vi "Setup_Environment.vi"() -> (0 "First Time":bool)   [LabVIEW 2022 SP3]
uses:
  File/Setup_Filetype.ctl
  Globals/Meas_global.vi
panel:
  out "error string":string
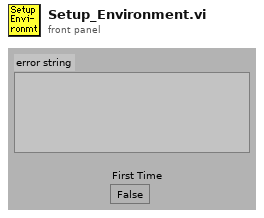
[diagram p1: front panel]
types:
  T1 = typedef "Setup_Filetype.ctl" = enum16{"Measurement Setups", "Calibration Setups", "General", "Results File Plotter Setups", "Speed Calib Tweaks"}
  T2 = cluster{"Start Index":i32, "End Index":i32, "Smoothing":enum16{"Linear", "Logarithmic"}, "Number of smoothed estimates":i32, "X axis":cluster{"Mapping":u16, "Format":u16}, "Y axis":cluster{"Mapping":u16, "Format":u16}, "Use Whole Input Array?":bool}[]
  T3 = cluster{"Start Index":i32, "End Index":i32, "Smoothing":enum16{"Linear", "Logarithmic"}, "Number of smoothed estimates":i32, "X axis":cluster{"Mapping":u16, "Format":u16}, "Y axis":cluster{"Mapping":u16, "Format":u16}, "Use Whole Input Array?":bool}
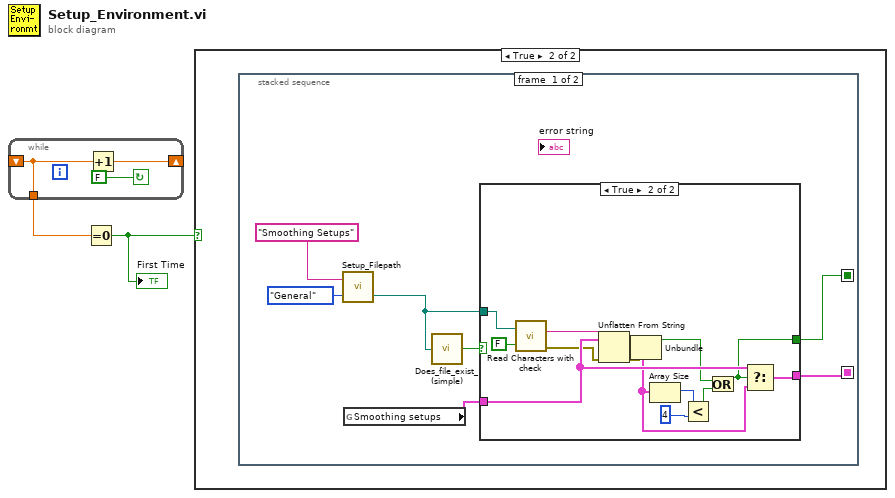
[diagram p0: block diagram]
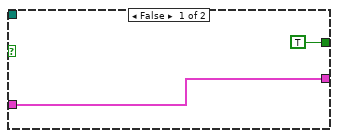
[diagram p3: hidden frame]
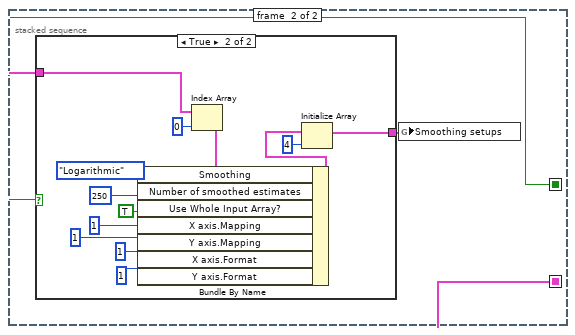
[diagram p4: hidden frame]
diagram:
  n1 = while {
    tunnel: [w5] -> w2
    shift-left: _ -> [w5]
    shift-right: [w4] -> _
    stop <- FALSE continue-if-true
    n2 = Increment(x=w5) -> (x+1=w4:dbl)
  }
  n3 = Equal To 0?(x=w2) -> (x = 0?=w1:bool)
  "First Time" <- w1
  n4 = case shown="True" w1 {
    frame False {
    }
    frame True {
      n5 = stacked-sequence {
        seq-local: [w10 _] -> [_ w30]
        seq-local: [w9 _] -> [_ w29]
        frame #0 {
          n6 = call "Setup_Filepath.vi"("Setup File Type"=Setup_Filetype."General", "Filename in"="Smoothing Setups" ("Substring")) -> ("Filename Out"=w6:path)  [unwired: 1 out]
          n7 = global read "Meas_global.vi" "Smoothing setups"() -> (w11:T2)
          n8 = call "Does_file_exist_(simple).vi"("Pathname"=w6) -> ("exists?"=w12:bool)
          n9 = case shown="True" w12 {
            tunnel: w6 -> [_ w18]
            tunnel: w11 -> [w14 w27]
            tunnel: [TRUE ("err") w20] -> w10
            tunnel: [w14 w26] -> w9
            frame False {
            }
            frame True {
              n10 = call "Read Characters with check.vi"("Call EnFlo Error Handler?"=FALSE, "file (use dialog)"=w18) -> ("error out"=w16:errorcluster, "Read String"=w17:string)
              n11 = Unflatten From String(type=w27, binary string=w17, error in (no error)=w16) -> (value=w21:T2, error out=w19:errorcluster)  [unwired: 3 out]
              n12 = Unbundle(w19) -> ("status"=w22:bool)  [unwired: 2 out]
              n13 = Array Size(array=w21) -> (size(s)=w25:i32)
              n14 = Less?(x=w25, y=4) -> (x < y?=w23:bool)
              n15 = Or(x=w22, y=w23) -> (x .or. y?=w20:bool)
              n16 = Select(t=w27, s=w20, f=w21) -> (s? t:f=w26:T2)
            }
          }
        }
        frame #1 {
          n17 = case shown="True" w30 {
            tunnel: [w31 w41] -> w28
            tunnel: w29 -> [w31 w34]
            frame False {
            }
            frame True {
              n18 = Index Array(array=w34, index=0 ("Index")) -> (element=w42:T3)
              n19 = Bundle By Name(cluster=w42, "Smoothing"=enum16{"Linear", "Logarithmic"}."Logarithmic" ("Bundle Element"), "Number of smoothed estimates"=250 ("Bundle Element"), "Use Whole Input Array?"=TRUE ("Bundle Element"), "X axis.Mapping"=u16 1 ("Bundle Element"), "Y axis.Mapping"=u16 1 ("Bundle Element"), "X axis.Format"=u16 1 ("Bundle Element"), "Y axis.Format"=u16 1 ("Bundle Element")) -> (w35:T3)
              n20 = Initialize Array(w35, 4) -> (w41:T2)
            }
          }
          n21 = global write "Meas_global.vi" "Smoothing setups"(w28) -> ()
        }
      }
    }
  }
